vi "FormatButtonText.vi"(8 "TextColor":u32, 10 "TextBoxSize":T1, 11 "Button":refnum<vi>) -> ()   [LabVIEW 2018]
uses:
  <vilib>/Utility/miscctls.llb/LVBoundsTypeDef.ctl
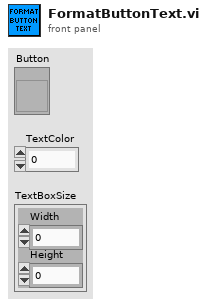
[diagram p1: front panel]
types:
  T1 = typedef "LVBoundsTypeDef.ctl" = cluster{"Width":u32, "Height":u32}
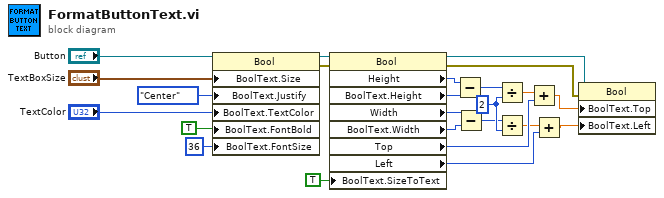
[diagram p0: block diagram]
diagram:
  w9 = u32 2 ("y")
  n1 = property on="Property Node" class="Bool"(reference="Button", "BoolText.Size"="TextBoxSize", "BoolText.Justify"=enum16{"Left", "Center", "Right"}."Center" ("Boolean Text.Justification"), "BoolText.TextColor"="TextColor", "BoolText.FontBold"=TRUE ("Boolean Text.Font:Bold"), "BoolText.FontSize"=u32 36 ("Boolean Text.Font:Size")) -> (reference out=w4:refnum<vi>, error out=w21:errorcluster)  [unwired: 1 in]
  n2 = property on="Property Node" class="Bool"(reference=w4, error in=w21, "BoolText.SizeToText"=TRUE ("Boolean Text.Size to Text?")) -> (reference out=w3:refnum<vi>, error out=w22:errorcluster, "Height"=w11:u32, "BoolText.Height"=w6:u32, "Width"=w13:u32, "BoolText.Width"=w10:u32, "Top"=w23:i32, "Left"=w24:i32)
  n3 = Subtract(x=w11, y=w6) -> (x-y=w7:u32)
  n4 = Subtract(x=w13, y=w10) -> (x-y=w8:u32)
  n5 = Divide(x=w7, y=w9) -> (x/y=w15:dbl)
  n6 = Divide(x=w8, y=w9) -> (x/y=w16:dbl)
  n7 = Add(x=w15, y=w23) -> (x+y=w12:dbl)
  n8 = Add(x=w16, y=w24) -> (x+y=w14:dbl)
  n9 = property on="Property Node" class="Bool"(reference=w3, error in=w22, "BoolText.Top"=w12, "BoolText.Left"=w14) -> ()  [unwired: 2 out]
